vi "motorFunction.vi"(0 "VISA Refnum in":refnum<visa-resource-name>, 1 "zone 3 co2":dbl min=0.0 max=100.0, 2 "Light 2":i32 min=0 max=1, 3 "zone 3 return":dbl min=0.0 max=100.0, 4 "Light 1":i32 min=0 max=1, 5 "zone 2 co2":dbl min=0.0 max=100.0, 6 "fresh air":dbl min=0.0 max=100.0, 7 "error in (no error)":errorcluster, 8 "Light 3":i32 min=0 max=1, 9 "zone 1 co2":dbl min=0.0 max=100.0, 10 "zone 2 return":dbl min=0.0 max=100.0, 11 "zone 3 inlet":dbl min=0.0 max=100.0, 12 "zone 2 inlet":dbl min=0.0 max=100.0, 13 "Fans":i32 min=0 max=1, 14 "zone 1 return":dbl min=0.0 max=100.0, 16 "zone 1 inlet":dbl min=0.0 max=100.0) -> (20 "VISA Refnum out":refnum<visa-resource-name>, 27 "error out":errorcluster)   [LabVIEW 2019]
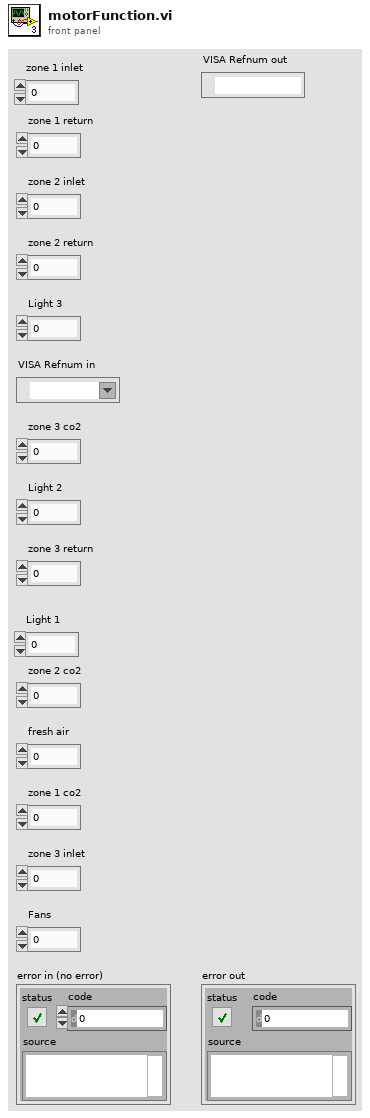
[diagram p1: front panel]
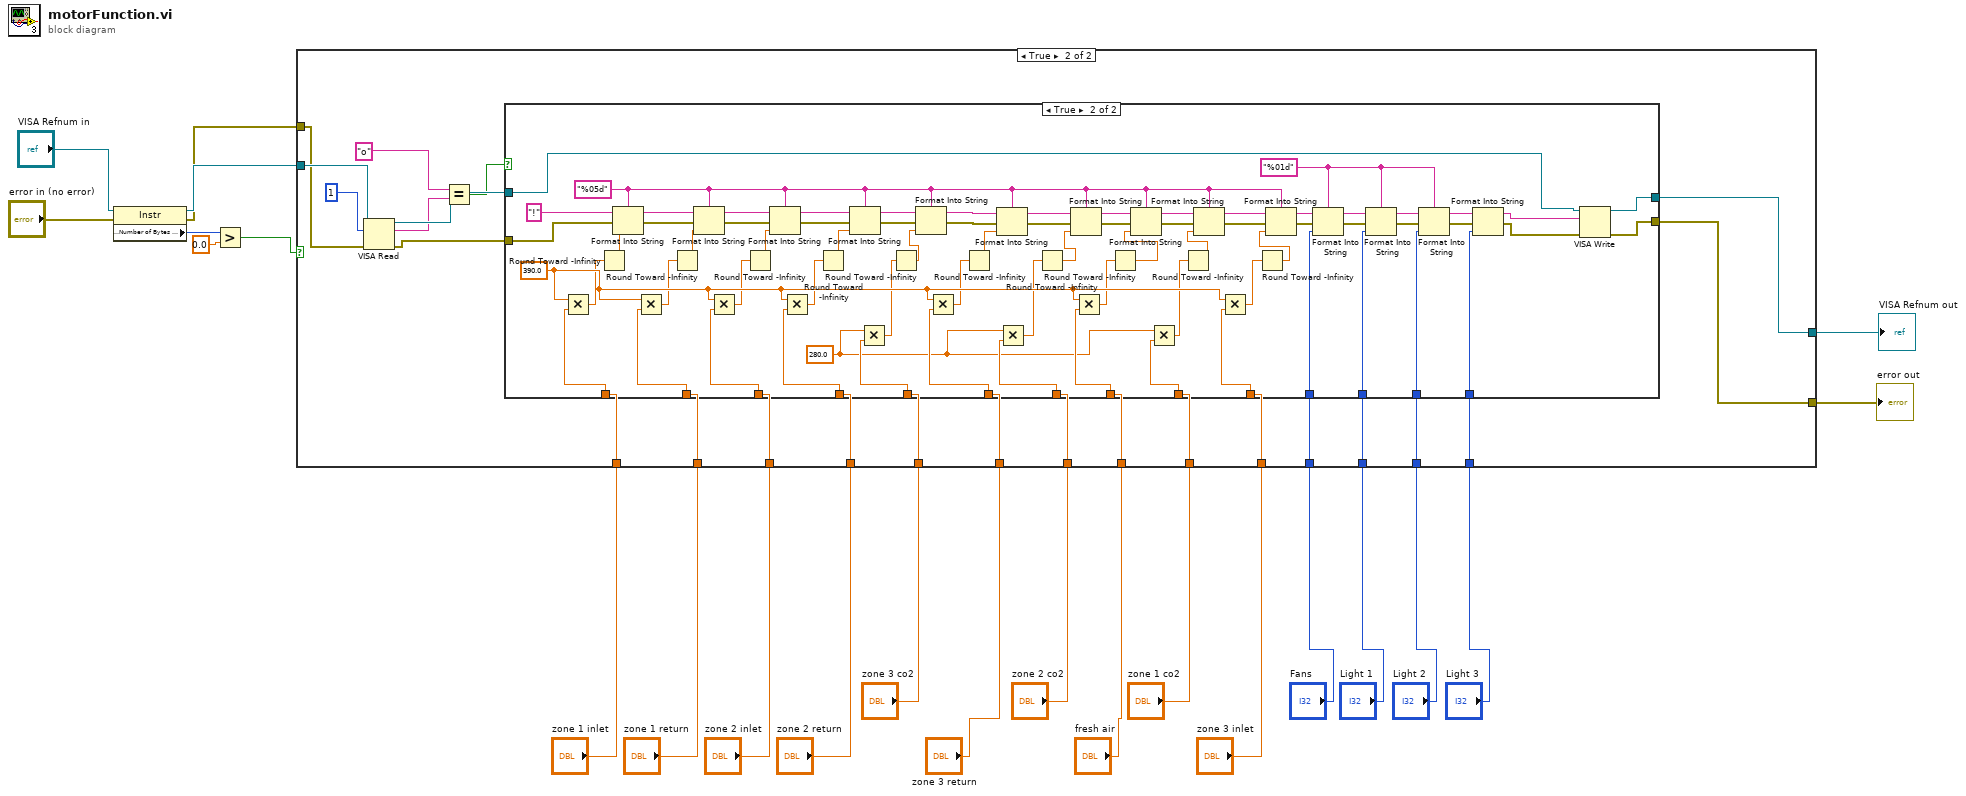
[diagram p0: block diagram]
diagram:
  n1 = property class="Instr"(reference="VISA Refnum in", error in="error in (no error)") -> (reference out=w4:refnum<visa-resource-name>, error out=w3:errorcluster, "Serial Settings:Number of Bytes at Serial Port"=w6:u32)
  n2 = Greater?(x=w6, y=0.0) -> (0:w5:bool)
  n3 = case shown="True" w5 {
    tunnel: [w24 w48] -> w23
    tunnel: [w25 w47] -> w22
    tunnel: "Light 3" -> [_ w44]
    tunnel: "Light 2" -> [_ w43]
    tunnel: "Light 1" -> [_ w42]
    tunnel: "Fans" -> [_ w41]
    tunnel: "zone 3 inlet" -> [_ w40]
    tunnel: "zone 1 co2" -> [_ w39]
    tunnel: "fresh air" -> [_ w38]
    tunnel: "zone 2 co2" -> [_ w37]
    tunnel: "zone 3 return" -> [_ w36]
    tunnel: "zone 3 co2" -> [_ w35]
    tunnel: "zone 2 return" -> [_ w34]
    tunnel: "zone 2 inlet" -> [_ w33]
    tunnel: "zone 1 inlet" -> [_ w29]
    tunnel: "zone 1 return" -> [_ w28]
    tunnel: w4 -> [w24 w27]
    tunnel: w3 -> [w25 w26]
    frame False {
    }
    frame True {
      n4 = VISA Read(VISA resource name=w27, byte count=u32 1, error in (no error)=w26) -> (VISA resource name out=w49:refnum<visa-resource-name>, read buffer=w31:string, error out=w46:errorcluster)  [unwired: 1 out]
      n5 = Equal?(x="o" ("y"), y=w31) -> (x = y?=w45:bool)
      n6 = case shown="True" w45 {
        tunnel: [w50 w107] -> w48
        tunnel: [w51 w106] -> w47
        tunnel: w29 -> [_ w83]
        tunnel: w28 -> [_ w82]
        tunnel: w33 -> [_ w81]
        tunnel: w34 -> [_ w80]
        tunnel: w35 -> [_ w79]
        tunnel: w36 -> [_ w78]
        tunnel: w37 -> [_ w77]
        tunnel: w38 -> [_ w76]
        tunnel: w39 -> [_ w75]
        tunnel: w40 -> [_ w74]
        tunnel: w41 -> [_ w90]
        tunnel: w42 -> [_ w89]
        tunnel: w43 -> [_ w88]
        tunnel: w44 -> [_ w87]
        tunnel: w46 -> [w51 w86]
        tunnel: w49 -> [w50 w85]
        frame False {
        }
        frame True {
          w52 = 280.0 ("x")
          w73 = 390.0 ("y")
          w94 = "%01d" ("format string")
          w101 = "%05d" ("format string")
          n7 = Multiply(x=w73, y=w83) -> (x*y=w53:dbl)
          n8 = Round Toward -Infinity(1:w53) -> (0:w72:dbl)
          n9 = Format Into String(format string=w101, initial string="!" ("write buffer"), error in=w86, w72) -> (resulting string=w121:string, error out=w122:errorcluster)
          n10 = Multiply(x=w73, y=w82) -> (x*y=w54:dbl)
          n11 = Round Toward -Infinity(1:w54) -> (0:w71:dbl)
          n12 = Format Into String(format string=w101, initial string=w121, error in=w122, w71) -> (resulting string=w119:string, error out=w120:errorcluster)
          n13 = Multiply(x=w73, y=w81) -> (x*y=w55:dbl)
          n14 = Round Toward -Infinity(1:w55) -> (0:w70:dbl)
          n15 = Format Into String(format string=w101, initial string=w119, error in=w120, w70) -> (resulting string=w117:string, error out=w118:errorcluster)
          n16 = Multiply(x=w73, y=w80) -> (x*y=w56:dbl)
          n17 = Round Toward -Infinity(1:w56) -> (0:w69:dbl)
          n18 = Format Into String(format string=w101, initial string=w117, error in=w118, w69) -> (resulting string=w115:string, error out=w116:errorcluster)
          n19 = Multiply(x=w52, y=w79) -> (x*y=w57:dbl)
          n20 = Round Toward -Infinity(1:w57) -> (0:w68:dbl)
          n21 = Format Into String(format string=w101, initial string=w115, error in=w116, w68) -> (resulting string=w113:string, error out=w114:errorcluster)
          n22 = Multiply(x=w73, y=w78) -> (x*y=w58:dbl)
          n23 = Round Toward -Infinity(1:w58) -> (0:w67:dbl)
          n24 = Format Into String(format string=w101, initial string=w113, error in=w114, w67) -> (resulting string=w111:string, error out=w112:errorcluster)
          n25 = Multiply(x=w52, y=w77) -> (x*y=w59:dbl)
          n26 = Round Toward -Infinity(1:w59) -> (0:w66:dbl)
          n27 = Format Into String(format string=w101, initial string=w111, error in=w112, w66) -> (resulting string=w110:string, error out=w109:errorcluster)
          n28 = Multiply(x=w73, y=w76) -> (x*y=w60:dbl)
          n29 = Round Toward -Infinity(1:w60) -> (0:w65:dbl)
          n30 = Format Into String(format string=w101, initial string=w110, error in=w109, w65) -> (resulting string=w103:string, error out=w105:errorcluster)
          n31 = Multiply(x=w52, y=w75) -> (x*y=w61:dbl)
          n32 = Round Toward -Infinity(1:w61) -> (0:w64:dbl)
          n33 = Format Into String(format string=w101, initial string=w103, error in=w105, w64) -> (resulting string=w102:string, error out=w104:errorcluster)
          n34 = Multiply(x=w73, y=w74) -> (x*y=w62:dbl)
          n35 = Round Toward -Infinity(1:w62) -> (0:w63:dbl)
          n36 = Format Into String(format string=w101, initial string=w102, error in=w104, w63) -> (resulting string=w97:string, error out=w100:errorcluster)
          n37 = Format Into String(format string=w94, initial string=w97, error in=w100, w90) -> (resulting string=w96:string, error out=w99:errorcluster)
          n38 = Format Into String(format string=w94, initial string=w96, error in=w99, w89) -> (resulting string=w95:string, error out=w98:errorcluster)
          n39 = Format Into String(format string=w94, initial string=w95, error in=w98, w88) -> (resulting string=w92:string, error out=w93:errorcluster)
          n40 = Format Into String(initial string=w92, error in=w93, w87) -> (resulting string=w84:string, error out=w91:errorcluster)  [unwired: 1 in]
          n41 = VISA Write(VISA resource name=w85, write buffer=w84, error in (no error)=w91) -> (VISA resource name out=w107:refnum<visa-resource-name>, error out=w106:errorcluster)  [unwired: 1 out]
        }
      }
    }
  }
  "VISA Refnum out" <- w23
  "error out" <- w22
